vi "owntest.vi"() -> ()   [LabVIEW 2019]
panel:
  out "Array 5":i32[][](array[numeric])
  out "Array 4":i32[](array[numeric])
  out "Output Tunnel Result (Last Value)":i32
  out "Output Tunnel Result 2":i32[](array[numeric])
  in  "1D DBL Array Input 2":dbl[](array[numeric])=[25.0, 50.0, 75.0, 100.0, 125.0, 150.0, 175.0, 200.0, 225.0, 250.0, 275.0, 300.0]
  out "Input Tunnel Result (Auto Index) 2":dbl
  out "Current Iteration 2":i32
  out "Input Tunnel Result (Last Value)":dbl[](array[numeric])
  out "Output Tunnel Result":i32[](array[numeric])
  in  "1D DBL Array Input":dbl[](array[numeric])=[25.0, 50.0, 75.0, 100.0, 125.0, 150.0, 175.0, 200.0, 225.0, 250.0, 275.0, 300.0]
  out "Input Tunnel Result (Auto Index)":dbl
  out "Current Iteration":i32
  out "Array 3":i32[](array[numeric])
  out "Array 2":i32[](array[numeric])
  out "Numeric 9":i32
  out "Numeric 8":i32
  out "Numeric 6":i32
  out "Numeric 5":i32
  out "Numeric 4":i32
  out "Numeric 3":dbl
  in  "Array":dbl[](array[numeric])
  out "Waveform Graph":waveform(dbl)(graph)
  in  "Waveform":waveform(dbl)
  out "Numeric 2":i32
  out "Numeric":i32
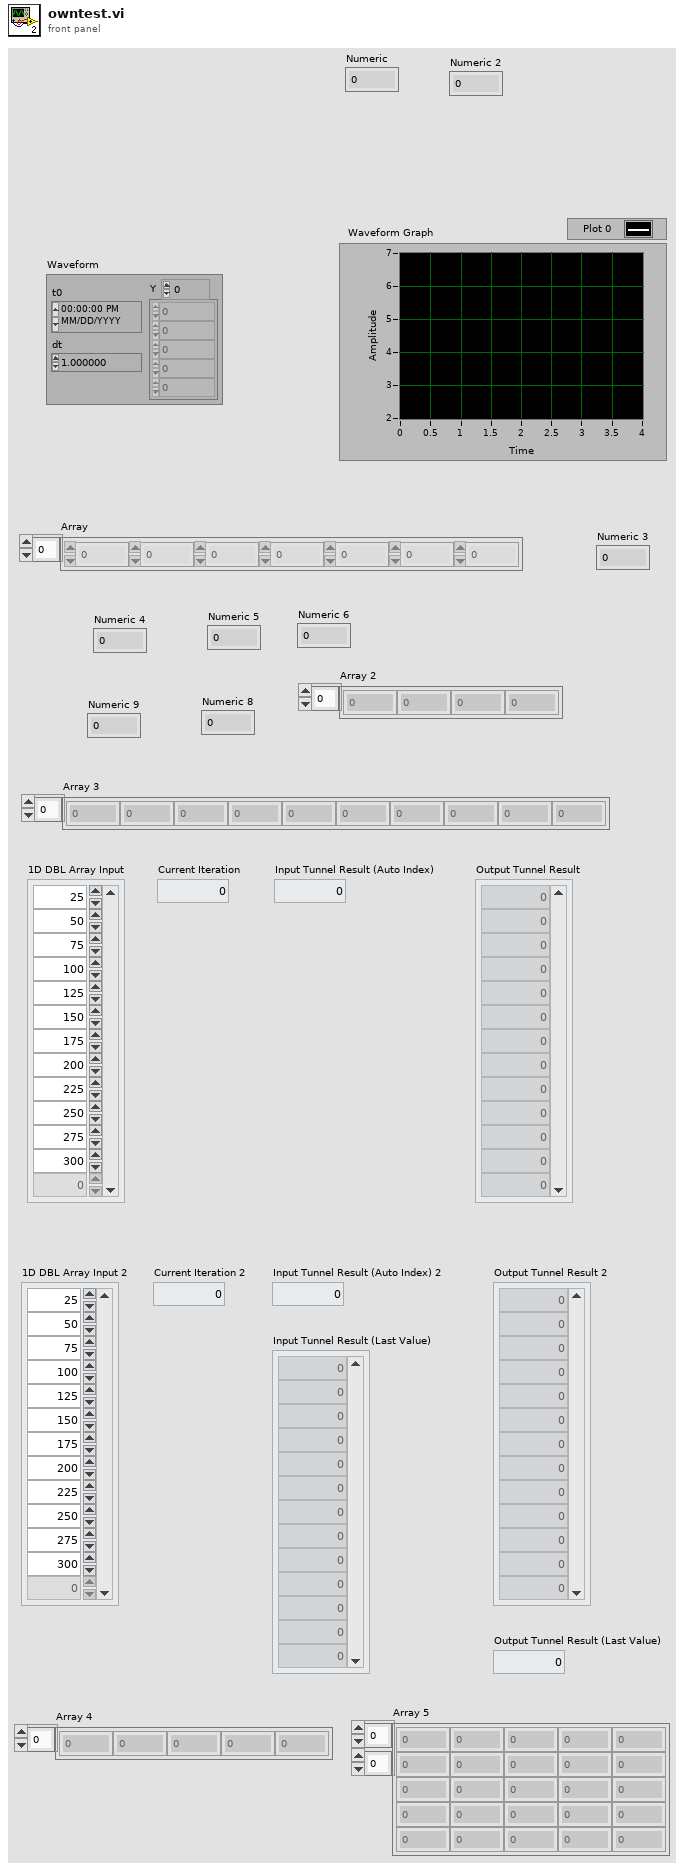
[diagram p1: front panel]
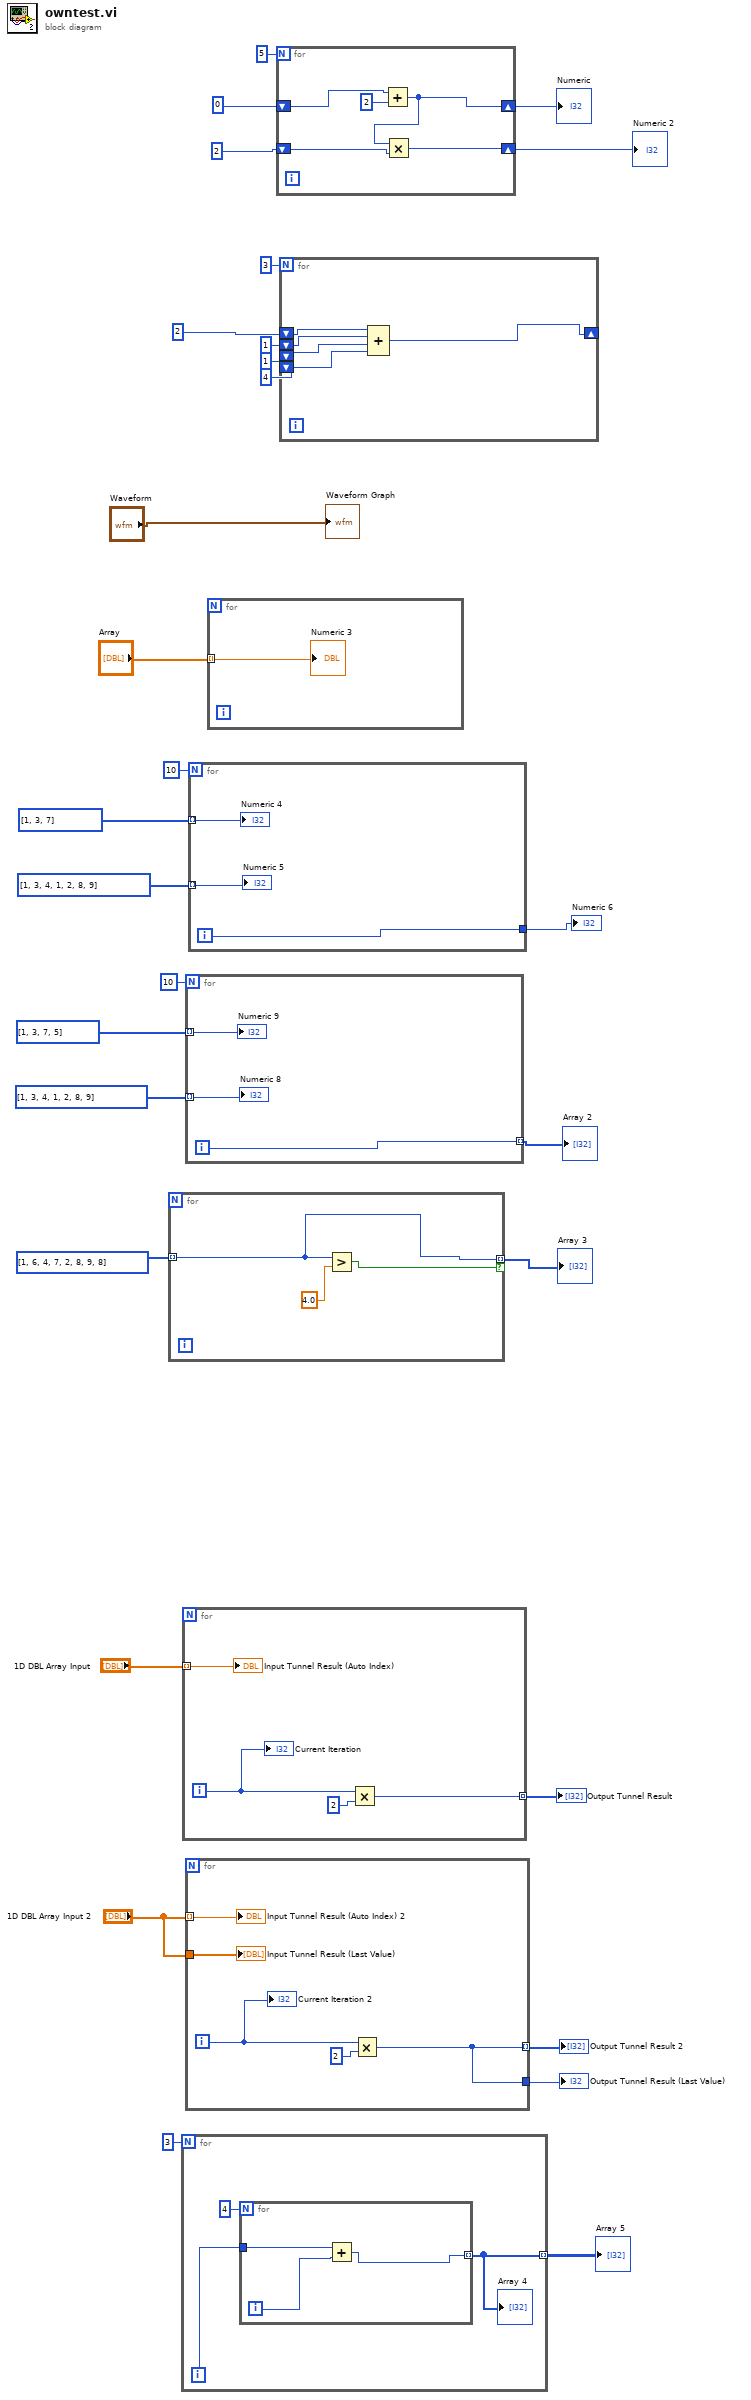
[diagram p0: block diagram]
diagram:
  n1 = for {
    tunnel: i32[] [1, 6, 4, 7, 2, 8, 9, 8] -> [w31] mode=indexing
    tunnel: [w31] -> w8 mode=indexing if=w30
    n2 = Greater?(x=w31, y=4.0) -> (0:w30:bool)
  }
  "Array 3" <- w8
  n3 = for {
    N: 3 -> [_]
    tunnel: [w33] -> w1 mode=indexing
    i -> [w34]
    n4 = for {
      N: 4 -> [_]
      tunnel: w34 -> [w37]
      tunnel: [w36] -> w33 mode=indexing
      i -> [w38]
      n5 = Add(x=w37, y=w38) -> (x+y=w36:i32)
    }
    "Array 4" <- w33
  }
  "Array 5" <- w1
  n6 = for {
    tunnel: "1D DBL Array Input" -> [w40] mode=indexing
    tunnel: [w39] -> w6 mode=indexing
    i -> [w42]
    n7 = Multiply(x=w42, y=2) -> (x*y=w39:i32)
    "Input Tunnel Result (Auto Index)" <- w40
    "Current Iteration" <- w42
  }
  "Output Tunnel Result" <- w6
  n8 = for {
    N: 10 -> [_]
    tunnel: i32[] [1, 3, 7, 5] -> [w45] mode=indexing
    tunnel: i32[] [1, 3, 4, 1, 2, 8, 9] -> [w44] mode=indexing
    tunnel: [w43] -> w10 mode=indexing
    i -> [w43]
    "Numeric 9" <- w45
    "Numeric 8" <- w44
  }
  "Array 2" <- w10
  n9 = for {
    tunnel: "1D DBL Array Input 2" -> [w48] mode=indexing
    tunnel: [w46] -> w5 mode=indexing
    tunnel: "1D DBL Array Input 2" -> [w47]
    tunnel: [w46] -> w3
    i -> [w50]
    n10 = Multiply(x=w50, y=2) -> (x*y=w46:i32)
    "Input Tunnel Result (Auto Index) 2" <- w48
    "Current Iteration 2" <- w50
    "Input Tunnel Result (Last Value)" <- w47
  }
  "Output Tunnel Result 2" <- w5
  "Output Tunnel Result (Last Value)" <- w3
  n11 = for {
    N: 10 -> [_]
    tunnel: i32[] [1, 3, 7] -> [w53] mode=indexing
    tunnel: i32[] [1, 3, 4, 1, 2, 8, 9] -> [w52] mode=indexing
    tunnel: [w51] -> w14
    i -> [w51]
    "Numeric 4" <- w53
    "Numeric 5" <- w52
  }
  "Numeric 6" <- w14
  n12 = for {
    tunnel: "Array" -> [w54] mode=indexing
    "Numeric 3" <- w54
  }
  n13 = for {
    N: 5 -> [_]
    shift-right: [w56] -> w26
    shift-left: 0 -> [w59]
    shift-right: [w57] -> w25
    shift-left: 2 -> [w55]
    n14 = Add(x=w59, y=2) -> (x+y=w56:i32)
    n15 = Multiply(x=w56, y=w55) -> (x*y=w57:i32)
  }
  "Numeric" <- w26
  "Numeric 2" <- w25
  n16 = for {
    N: 3 -> [_]
    shift-right: [w63] -> _
    shift-left: 2 -> [w64]
    shift-left: 1 -> [w62]
    shift-left: 1 -> [w61]
    shift-left: 4 -> [w60]
    n17 = Compound Arithmetic op=ADD(w64, w62, w61, w60) -> (w63:i32)
  }
  "Waveform Graph" <- "Waveform"
